vi "Get Tuner Type.vi"(8 "error in (no error)":errorcluster, 11 "RTL-SDR in":refnum<class "Session.lvclass">) -> (0 "error out":errorcluster, 2 "Tuner Type":T1, 3 "RTL-SDR out":refnum<class "Session.lvclass">)   [LabVIEW 2020, in "RTL-SDR.lvlib" / "Session.lvclass"]
uses:
  Session.lvclass
  Tuner Type.ctl
  RTL-SDR.lvlib
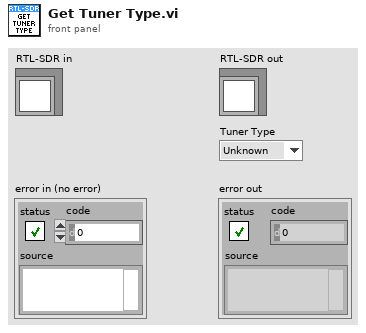
[diagram p1: front panel]
types:
  T1 = typedef "RTL-SDR.lvlib/Tuner Type.ctl" = enum32{"Unknown", "E4000", "FC0012", "FC0013", "FC2580", "R820T", "R828D"}
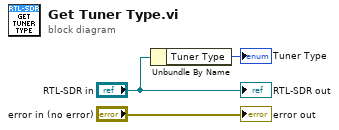
[diagram p0: block diagram]
diagram:
  n1 = Unbundle By Name("RTL-SDR in") -> ("Tuner Type"=→"Tuner Type":T1)
  "error out" <- "error in (no error)"
  "RTL-SDR out" <- "RTL-SDR in"
